vi "While_Loop.vi"() -> ()   [LabVIEW 2022 SP3]
panel:
  out "Numeric 2":i32
  out "Waveform Chart":dbl(graph)
  out "Boolean":bool
  out "Numeric":i32
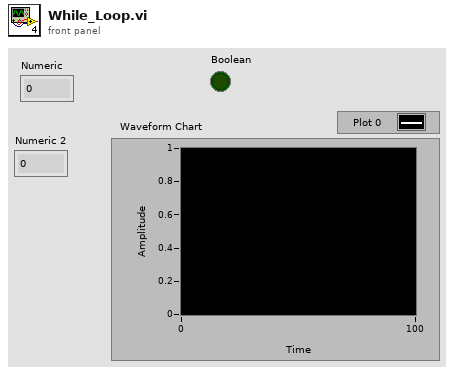
[diagram p1: front panel]
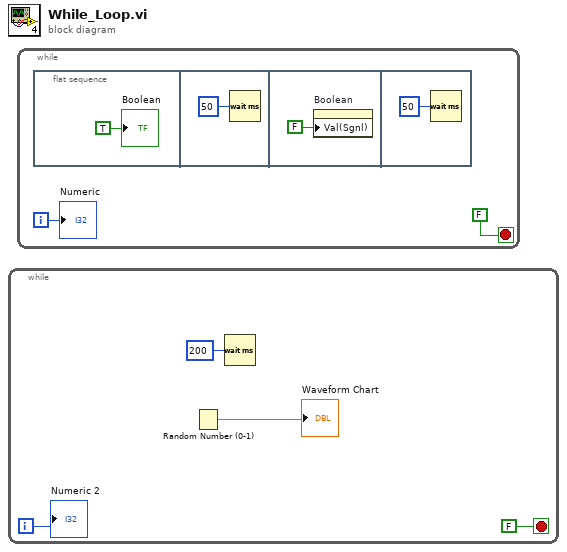
[diagram p0: block diagram]
diagram:
  n1 = while {
    i -> [w1]
    stop <- FALSE stop-if-true
    n2 = Random Number (0-1)() -> (number: 0 to 1=→"Waveform Chart":dbl)
    n3 = Wait (ms)(milliseconds to wait=u32 200) -> ()  [unwired: 1 out]
    "Numeric 2" <- w1
  }
  n4 = while {
    i -> [w6]
    stop <- FALSE stop-if-true
    n5 = flat-sequence {
      frame #0 {
        "Boolean" <- TRUE ("Boolean")
      }
      frame #1 {
        n6 = Wait (ms)(milliseconds to wait=u32 50) -> ()  [unwired: 1 out]
      }
      frame #2 {
        n7 = property on="Boolean" class="Bool (strict)"("Val(Sgnl)"=FALSE ("Value (Signaling)")) -> ()  [unwired: 2 in, 2 out]
      }
      frame #3 {
        n8 = Wait (ms)(milliseconds to wait=u32 50) -> ()  [unwired: 1 out]
      }
    }
    "Numeric" <- w6
  }
